vi "WristEncoder.vi"(1 "Terms":i32) -> ()   [LabVIEW 2017]
uses:
  Phoenix-LabVIEW/Motor Controller/Get/CTRE_Phoenix_MotorController_GetSelectedSensorData.vi
  Robot Global Data.vi
panel:
  out "Position":dbl(graph)
  out "Velocity":dbl(graph)
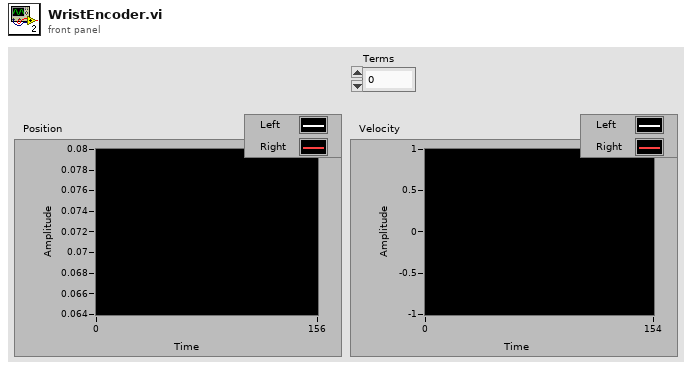
[diagram p1: front panel]
types:
  T1 = typedef "WPI_MotorControlDeviceRef.ctl" = cluster{"DeviceStatus":errorcluster, "Type":T2, "PWM":cluster{"PWM Channel":T3, "DeadBand":T4}, "CAN":cluster{"Device Number":u8, "SetOutput VI Ref":variant, "GetOutput VI Ref":variant, "Enable VI Ref":variant, "Disable VI Ref":variant, "Data":variant}, "Invert":bool, "DIO PWM":cluster{"PWM \"Enable\" Channel":T3, "DIOChannel":T5, "PWM Rate":dbl}}
  T2 = typedef "WPI_MotorControlType.ctl" = enum16{"PWM", "CAN", "DIO PWM"}
  T3 = typedef "FPGA_DIOPWMChannel.ctl" = enum8{"PWM 0", "PWM 1", "PWM 2", "PWM 3", "PWM 4", "PWM 5", "PWM 6", "PWM 7", "PWM 8", "PWM 9", "PWM MXP 0", "PWM MXP 1", "PWM MXP 2", "PWM MXP 3", "PWM MXP 4", "PWM MXP 5", "PWM MXP 6", "PWM MXP 7", "PWM MXP 8", "PWM MXP 9", "Invalid"}
  T4 = typedef "WPI_PWMDeadband.ctl" = cluster{"Name":string, "maxPositivePwm":i32, "minPositivePwm":i32, "centerPwm":i32, "maxNegativePwm":i32, "minNegativePwm":i32, "angularRange":u16}
  T5 = typedef "FPGA_DIOChannel.ctl" = enum8{"DIO 0", "DIO 1", "DIO 2", "DIO 3", "DIO 4", "DIO 5", "DIO 6", "DIO 7", "DIO 8", "DIO 9", "DIO MXP 0", "DIO MXP 1", "DIO MXP 2", "DIO MXP 3", "DIO MXP 4", "DIO MXP 5", "DIO MXP 6", "DIO MXP 7", "DIO MXP 8", "DIO MXP 9", "DIO MXP 10", "DIO MXP 11", "DIO MXP 12", "DIO MXP 13", "DIO MXP 14", "DIO MXP 15", "SPI Port CS1", "SPI Port CS2", "SPI Port CS3", "SPI Port MISO", "SPI Port MOSI", "Invalid"}
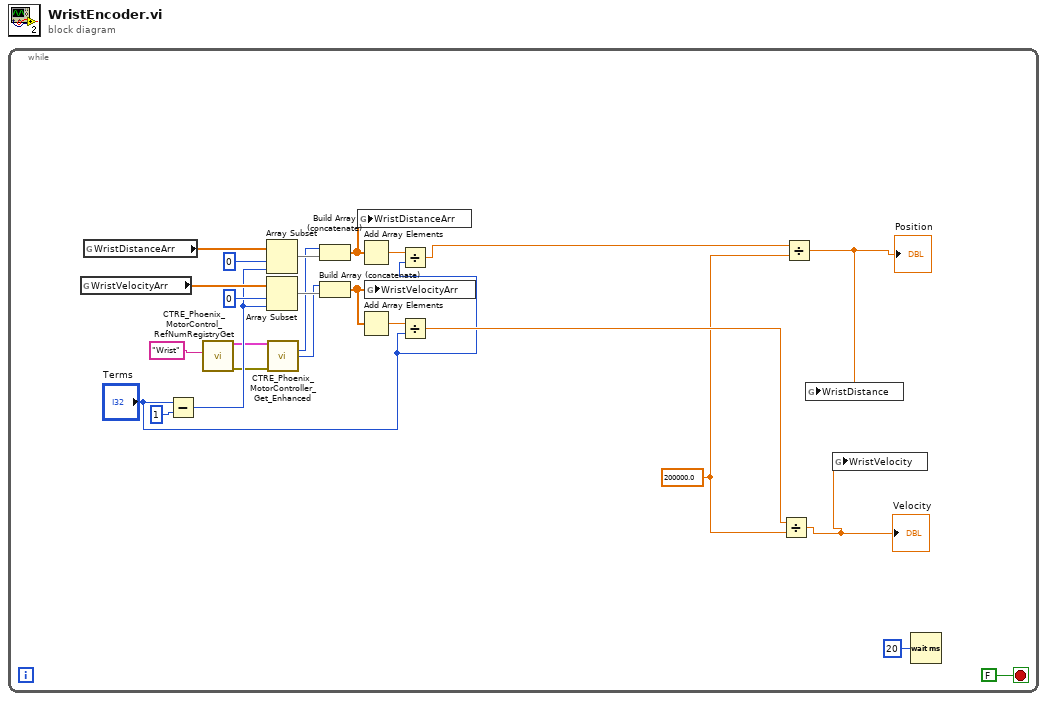
[diagram p0: block diagram]
diagram:
  n1 = while {
    stop <- FALSE stop-if-true
    w11 = 200000.0
    n2 = global read "Robot Global Data.vi" "WristVelocityArr"() -> (w23:dbl[])
    n3 = global read "Robot Global Data.vi" "WristDistanceArr"() -> (w25:dbl[])
    n4 = Subtract(x="Terms", y=1) -> (x-y=w19:i32)
    n5 = call "CTRE_Phoenix_MotorControl_RefNumRegistryGet.vi"("refnum name"="Wrist") -> ("error out"=w4:errorcluster, "PhoenixMotorControlDevRef"=w3:T1)  [unwired: 9 in]
    n6 = Array Subset(array=w25, index=0, length=w19) -> (w21:dbl[])
    n7 = Array Subset(array=w23, index=0, length=w19) -> (w18:dbl[])
    n8 = call-poly "CTRE_Phoenix_MotorController_Get_Enhanced.vi"("PhoenixMotorControlDevRef"=w3, "error in"=w4) -> ("Position (Raw Sensor Units)"=w1:i32, "Velocity (Raw Sensor Units per 100 ms)"=w2:i32)  [unwired: 10 in, 2 out]
    n9 = Build Array (concatenate)(w1, w21) -> (w17:dbl[])
    n10 = Build Array (concatenate)(w2, w18) -> (w16:dbl[])
    n11 = global write "Robot Global Data.vi" "WristDistanceArr"(w17) -> ()
    n12 = Add Array Elements(numeric array=w17) -> (sum=w15:dbl)
    n13 = Add Array Elements(numeric array=w16) -> (sum=w14:dbl)
    n14 = global write "Robot Global Data.vi" "WristVelocityArr"(w16) -> ()
    n15 = Divide(x=w15, y="Terms") -> (x/y=w13:dbl)
    n16 = Divide(x=w14, y="Terms") -> (x/y=w12:dbl)
    n17 = Divide(x=w12, y=w11) -> (x/y=w6:dbl)
    "Velocity" <- w6
    n18 = Divide(x=w13, y=w11) -> (x/y=w7:dbl)
    "Position" <- w7
    n19 = global write "Robot Global Data.vi" "WristDistance"(w7) -> ()
    n20 = global write "Robot Global Data.vi" "WristVelocity"(w6) -> ()
    n21 = Wait (ms)(milliseconds to wait=u32 20) -> ()  [unwired: 1 out]
  }
